vi "SetBySetLocalData.vi"(9 "SetCounterIN":i32, 10 "IndexCounterIN":i32, 11 "DataIN":string[][](array[string])) -> (0 "Empty DataOUT":bool, 1 "DataOUT":string[][](array[string]), 2 "SetCounterOUT":i32, 3 "IndexCounterOUT":i32)   [LabVIEW 2019, in "DataLogger.lvclass"]
doc: "Set by Set local data"
uses:
  DataLogger.lvclass
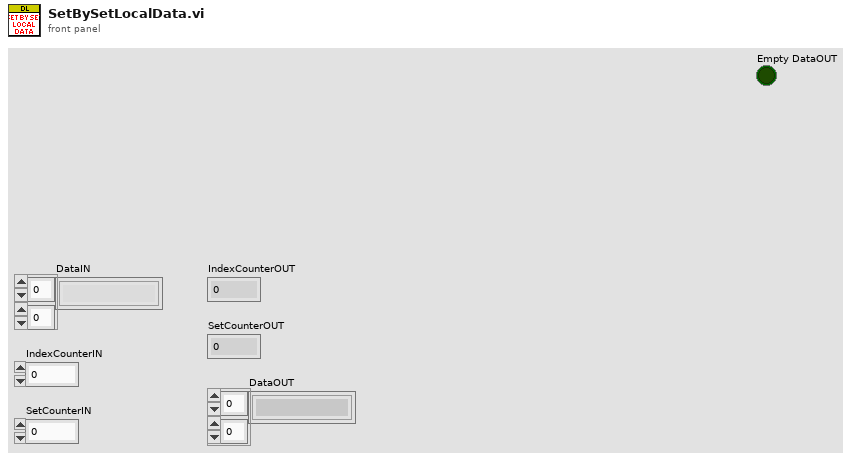
[diagram p1: front panel]
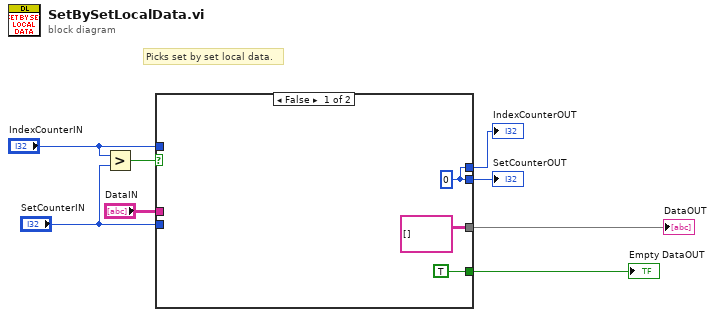
[diagram p0: block diagram]
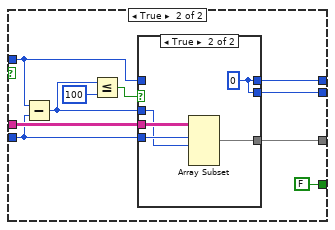
[diagram p2: hidden frame]
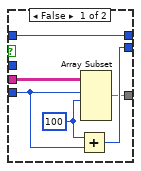
[diagram p3: hidden frame]
diagram:
  # "Picks set by set local data."
  n1 = Greater?(x="IndexCounterIN", y="SetCounterIN") -> (0:w6:bool)
  n2 = case shown="False" w6 {
    tunnel: "IndexCounterIN" -> [_ w14]
    tunnel: "SetCounterIN" -> [_ w18]
    tunnel: "DataIN" -> [_ w19]
    tunnel: [w11 w16] -> w7
    tunnel: [w11 w13] -> w8
    tunnel: [string[][] [] w15] -> w2
    tunnel: [TRUE FALSE] -> w1
    frame False {
      w11 = 0 ("length")
    }
    frame True {
      n3 = Subtract(x=w14, y=w18) -> (x-y=w17:i32)
      n4 = Less Or Equal?(x=w17, y=100) -> (x <= y?=w20:bool)
      n5 = case shown="True" w20 {
        tunnel: w19 -> [w27 w32]
        tunnel: w18 -> [w25 w31]
        tunnel: w17 -> [_ w30]
        tunnel: [w26 w28] -> w16
        tunnel: [w23 w29] -> w15
        tunnel: w14 -> [w22 _]
        tunnel: [w22 w28] -> w13
        frame False {
          w24 = 100 ("length")
          n6 = Add(x=w24, y=w25) -> (x+y=w26:i32)
          n7 = Array Subset(array=w27, index (row)=w25, length (row)=w24) -> (w23:string[][])  [unwired: 2 in]
        }
        frame True {
          w28 = 0
          n8 = Array Subset(array=w32, index (row)=w31, length (row)=w30) -> (w29:string[][])  [unwired: 2 in]
        }
      }
    }
  }
  "DataOUT" <- w2
  "IndexCounterOUT" <- w8
  "SetCounterOUT" <- w7
  "Empty DataOUT" <- w1
